vi "testLoadStamp.vi"() -> ()   [LabVIEW 2017]
uses:
  Gantry/Shared Components/Gantry Class/Gantry.lvclass
  Gantry/Shared Components/Gantry Class/Type Definitions/Virtual Modes.ctl
  Gantry/Shared Components/FlexWorktable/FlexWorktable.lvclass
panel:
  out "error out":errorcluster
  in  "Config Folder":path=path "C:/Users/husker/Desktop/gantry/Config"
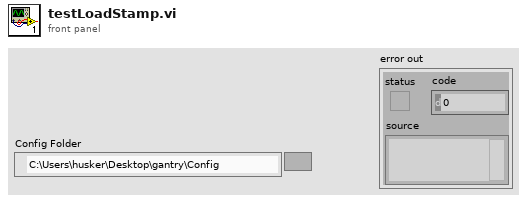
[diagram p1: front panel]
types:
  T1 = typedef "Virtual Modes.ctl" = enum16{"Nonvirtual", "Virtual"}
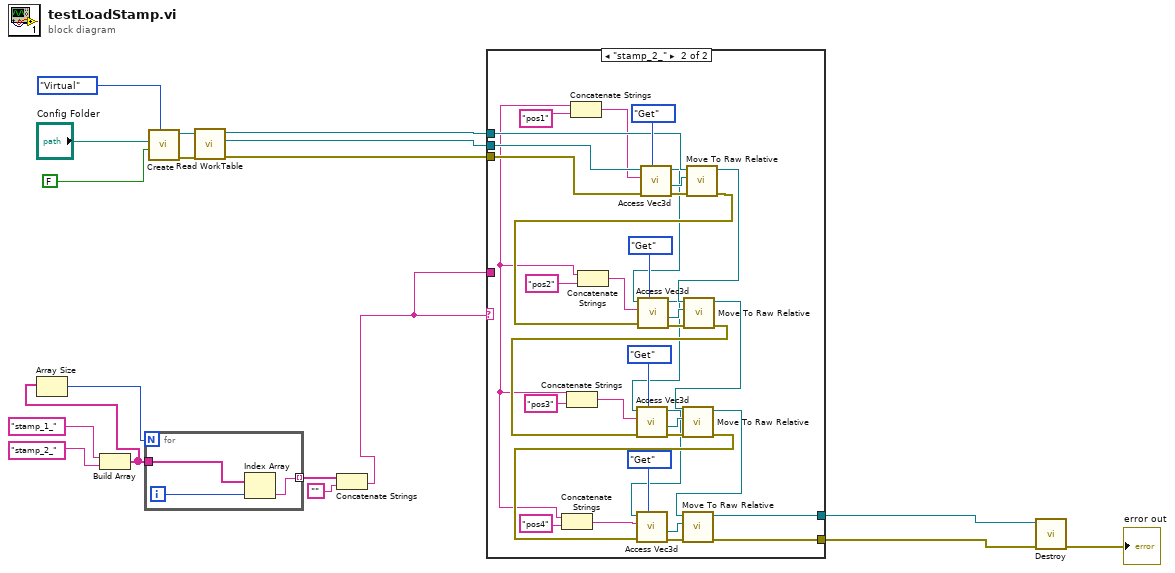
[diagram p0: block diagram]
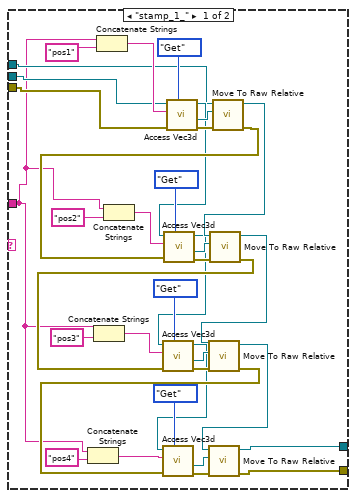
[diagram p2: hidden frame]
diagram:
  n1 = Build Array("stamp_1_", "stamp_2_") -> (w4:string[])
  n2 = Array Size(array=w4) -> (size(s)=w5:i32)
  n3 = for {
    N: w5 -> [_]
    tunnel: [w19] -> w3 mode=indexing
    tunnel: w4 -> [w21]
    i -> [w20]
    n4 = Index Array(array=w21, index=w20) -> (element=w19:string)
  }
  n5 = call "Create.vi"("Virtual Mode"=Virtual_Modes."Virtual", "HOME?"=FALSE, "Config Folder"="Config Folder") -> ("error out"=w13:errorcluster, "Gantry out"=w14:refnum<class "Gantry.lvclass">)  [unwired: 6 in, 1 out]
  n6 = call-dynamic "Read WorkTable.vi"("error in"=w13, "Gantry Class in"=w14) -> ("error out"=w10:errorcluster, "Worktable"=w12:refnum<class "FlexWorktable.lvclass">, "Gantry Class out"=w11:refnum<class "Gantry.lvclass">)  [unwired: 7 in]
  n7 = Concatenate Strings(w3, "") -> (w1:string)
  n8 = case shown="\"stamp_2_\"" w1 {
    tunnel: w12 -> [w24 w79]
    tunnel: w11 -> [w23 w78]
    tunnel: w10 -> [w25 w77]
    tunnel: [w27 w67] -> w9
    tunnel: [w26 w66] -> w8
    tunnel: w1 -> [w22 _]
    frame "stamp_1_" {
      n9 = Concatenate Strings(w22, "pos4" ("string")) -> (w31:string)
      n10 = Concatenate Strings(w22, "pos3" ("string")) -> (w33:string)
      n11 = Concatenate Strings(w22, "pos1" ("string")) -> (w29:string)
      n12 = Concatenate Strings(w22, "pos2" ("string")) -> (w34:string)
      n13 = call-dynamic "Access Vec3d.vi"("Get/Set"=enum16{"Get", "Set"}."Get", "error in (no error)"=w25, "Key"=w29, "FlexWorktable in"=w24) -> ("error out"=w55:errorcluster, "Value out"=w54:refnum<class "Vec3d.lvclass">, "FlexWorktable out"=w38:refnum<class "FlexWorktable.lvclass">)  [unwired: 5 in]
      n14 = call-dynamic "Move To Raw Relative.vi"("error in"=w55, "Delta"=w54, "Gantry in"=w23) -> ("error out"=w39:errorcluster, "Gantry out"=w44:refnum<class "Gantry.lvclass">)  [unwired: 7 in]
      n15 = call-dynamic "Access Vec3d.vi"("Get/Set"=enum16{"Get", "Set"}."Get", "error in (no error)"=w39, "Key"=w34, "FlexWorktable in"=w38) -> ("error out"=w52:errorcluster, "Value out"=w51:refnum<class "Vec3d.lvclass">, "FlexWorktable out"=w37:refnum<class "FlexWorktable.lvclass">)  [unwired: 5 in]
      n16 = call-dynamic "Move To Raw Relative.vi"("error in"=w52, "Delta"=w51, "Gantry in"=w44) -> ("error out"=w42:errorcluster, "Gantry out"=w43:refnum<class "Gantry.lvclass">)  [unwired: 7 in]
      n17 = call-dynamic "Access Vec3d.vi"("Get/Set"=enum16{"Get", "Set"}."Get", "error in (no error)"=w42, "Key"=w33, "FlexWorktable in"=w37) -> ("error out"=w49:errorcluster, "Value out"=w48:refnum<class "Vec3d.lvclass">, "FlexWorktable out"=w36:refnum<class "FlexWorktable.lvclass">)  [unwired: 5 in]
      n18 = call-dynamic "Move To Raw Relative.vi"("error in"=w49, "Delta"=w48, "Gantry in"=w43) -> ("error out"=w40:errorcluster, "Gantry out"=w41:refnum<class "Gantry.lvclass">)  [unwired: 7 in]
      n19 = call-dynamic "Access Vec3d.vi"("Get/Set"=enum16{"Get", "Set"}."Get", "error in (no error)"=w40, "Key"=w31, "FlexWorktable in"=w36) -> ("error out"=w46:errorcluster, "Value out"=w45:refnum<class "Vec3d.lvclass">)  [unwired: 5 in, 1 out]
      n20 = call-dynamic "Move To Raw Relative.vi"("error in"=w46, "Delta"=w45, "Gantry in"=w41) -> ("error out"=w26:errorcluster, "Gantry out"=w27:refnum<class "Gantry.lvclass">)  [unwired: 7 in]
    }
    frame "stamp_2_" {
      n21 = Concatenate Strings("pos2" ("string")) -> (w64:string, w57:string)
      n22 = Concatenate Strings(w57, "pos4" ("string")) -> (w61:string)
      n23 = Concatenate Strings(w57, "pos3" ("string")) -> (w63:string)
      n24 = Concatenate Strings(w57, "pos1" ("string")) -> (w59:string)
      n25 = call-dynamic "Access Vec3d.vi"("Get/Set"=enum16{"Get", "Set"}."Get", "error in (no error)"=w77, "Key"=w59, "FlexWorktable in"=w79) -> ("error out"=w90:errorcluster, "Value out"=w89:refnum<class "Vec3d.lvclass">, "FlexWorktable out"=w70:refnum<class "FlexWorktable.lvclass">)  [unwired: 5 in]
      n26 = call-dynamic "Move To Raw Relative.vi"("error in"=w90, "Delta"=w89, "Gantry in"=w78) -> ("error out"=w71:errorcluster, "Gantry out"=w76:refnum<class "Gantry.lvclass">)  [unwired: 7 in]
      n27 = call-dynamic "Access Vec3d.vi"("Get/Set"=enum16{"Get", "Set"}."Get", "error in (no error)"=w71, "Key"=w64, "FlexWorktable in"=w70) -> ("error out"=w87:errorcluster, "Value out"=w86:refnum<class "Vec3d.lvclass">, "FlexWorktable out"=w69:refnum<class "FlexWorktable.lvclass">)  [unwired: 5 in]
      n28 = call-dynamic "Move To Raw Relative.vi"("error in"=w87, "Delta"=w86, "Gantry in"=w76) -> ("error out"=w74:errorcluster, "Gantry out"=w75:refnum<class "Gantry.lvclass">)  [unwired: 7 in]
      n29 = call-dynamic "Access Vec3d.vi"("Get/Set"=enum16{"Get", "Set"}."Get", "error in (no error)"=w74, "Key"=w63, "FlexWorktable in"=w69) -> ("error out"=w84:errorcluster, "Value out"=w83:refnum<class "Vec3d.lvclass">, "FlexWorktable out"=w68:refnum<class "FlexWorktable.lvclass">)  [unwired: 5 in]
      n30 = call-dynamic "Move To Raw Relative.vi"("error in"=w84, "Delta"=w83, "Gantry in"=w75) -> ("error out"=w72:errorcluster, "Gantry out"=w73:refnum<class "Gantry.lvclass">)  [unwired: 7 in]
      n31 = call-dynamic "Access Vec3d.vi"("Get/Set"=enum16{"Get", "Set"}."Get", "error in (no error)"=w72, "Key"=w61, "FlexWorktable in"=w68) -> ("error out"=w81:errorcluster, "Value out"=w80:refnum<class "Vec3d.lvclass">)  [unwired: 5 in, 1 out]
      n32 = call-dynamic "Move To Raw Relative.vi"("error in"=w81, "Delta"=w80, "Gantry in"=w73) -> ("error out"=w66:errorcluster, "Gantry out"=w67:refnum<class "Gantry.lvclass">)  [unwired: 7 in]
    }
  }
  n33 = call "Destroy.vi"("error in"=w8, "Gantry Class in"=w9) -> ("error out"=→"error out":errorcluster)  [unwired: 9 in]
